vi "2. String retrieve Rulers.vi"() -> ()   [LabVIEW 2017]
uses:
  d59d594f-6358-4fe9-a0ea-ade5f599e91a.vi
  177f037c-d6c1-4684-97ba-f775e359171c.vi
  f8914412-5770-4d7c-8ed9-34d3b6c64140.vi
  83982d16-e29d-493a-892c-93b6b063dd3a.vi
  40fc1cc9-77e3-4a14-9bb9-de70462c7f35.vi
  81b41104-5ca5-45e9-a143-87b761583821.vi
  38ed8c4c-bfe5-4ceb-af5c-8de10cee5e52.vi
  a345cc07-d10f-4275-8a18-17707c3f89e9.vi
  cabc4c38-4671-4b03-9489-31c074b0dc0c.vi
  efc68658-e21b-4998-9bfe-a9de0054dd82.vi
  0842be61-58c2-4c06-9355-20aaf40be817.vi
  a49a9376-e1ff-4fda-bff8-7fdb6b491f6f.vi
  API-String-Arugments-Support/_Support/Convert API String Arguments to Data(variant).vi
panel:
  out "output cluster 11":T1={"Empty API String"="", "2D DBL"=[[3.12, 4.113, 2.3, 5.0, 5.0, 2.3, 4.11, 5.0]], "Retrieved Data"=[[3.12, 4.113, 2.3, 5.0, 5.0, 2.3, 4.11, 5.0]]}
  out "output cluster 10":T2={"Empty API String"="", "Cluster Array"=[{"Name"="", "Child"={"Name"="ddd"}, "Bool"=FALSE}, {"Name"="ddd", "Child"={"Name"=""}, "Bool"=TRUE}], "Retrieved Data"=[{"Name"="", "Child"={"Name"="ddd"}, "Bool"=FALSE}, {"Name"="ddd", "Child"={"Name"=""}, "Bool"=TRUE}]}
  out "output cluster 9":T3={"Empty API String"="", "Cluster"={"Name"="abc", "Child"={"Name"="ddd"}, "Bool"=FALSE}, "Retrieved Data"={"Name"="abc", "Child"={"Name"="ddd"}, "Bool"=FALSE}}
  out "output cluster 8":T4={"Empty API String"="", "1D DBL"=[3.12, 4.11, 5.0], "Retrieved Data"=[3.12, 4.11, 5.0]}
  out "output cluster 7":T5={"Empty API String"="", "Enum"=enum."2 - bbbb", "Retrieved Data"=enum."1 - aaaa"}
  out "output cluster 6":T5
  out "output cluster 5":T6={"Empty API String"="", "Enum"=enum."ccccc", "Retrieved Data"=enum."aaaa"}
  out "output cluster 4":T7={"Empty API String"="", "DBL"=3.1415926, "Retrieved Data"=3.1415926}
  out "output cluster 3":T8={"Empty API String"="", "I32"=66, "Retrieved Data"=66}
  out "output cluster 2":T9={"Empty API String"="", "Boolean"=TRUE, "Retrieved Data"=TRUE}
  out "output cluster":T10={"Empty API String"="", "String"="abcd", "Retrieved Data"=""}
  out "output":T11={"Empty API String"="", "Path"=path "C:/ni-rt/data/a/2023.07.25", "Retrieved Data"=path "C:/ni-rt/data/a/2023.07.25"}
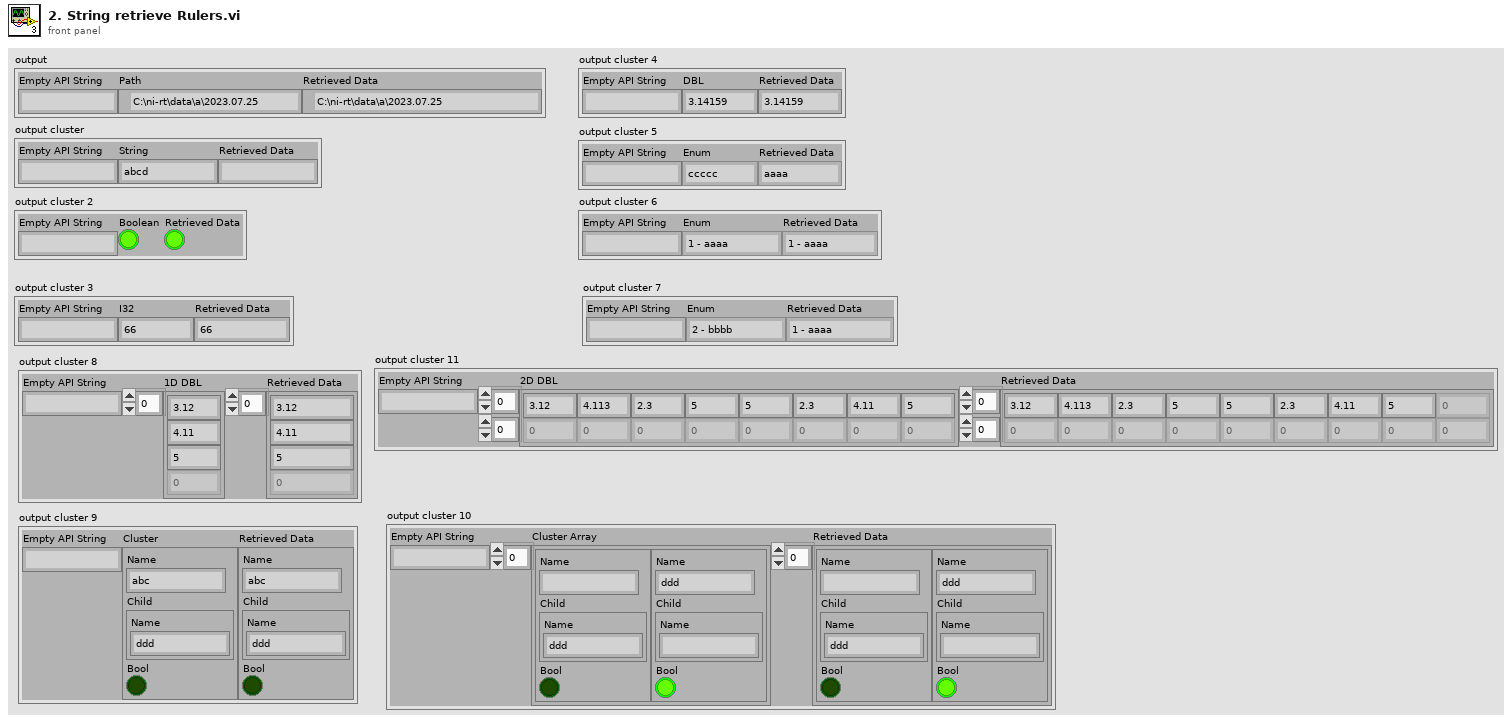
[diagram p1: front panel]
types:
  T1 = cluster{"Empty API String":string, "2D DBL":dbl[][], "Retrieved Data":dbl[][]}
  T2 = cluster{"Empty API String":string, "Cluster Array":cluster{"Name":string, "Child":cluster{"Name":string}, "Bool":bool}[], "Retrieved Data":cluster{"Name":string, "Child":cluster{"Name":string}, "Bool":bool}[]}
  T3 = cluster{"Empty API String":string, "Cluster":cluster{"Name":string, "Child":cluster{"Name":string}, "Bool":bool}, "Retrieved Data":cluster{"Name":string, "Child":cluster{"Name":string}, "Bool":bool}}
  T4 = cluster{"Empty API String":string, "1D DBL":dbl[], "Retrieved Data":dbl[]}
  T5 = cluster{"Empty API String":string, "Enum":enum16{"1 - aaaa", "2 - bbbb", "555 - ccccc"}, "Retrieved Data":enum16{"1 - aaaa", "2 - bbbb", "555 - ccccc"}}
  T6 = cluster{"Empty API String":string, "Enum":enum16{"aaaa", "bbbb", "ccccc"}, "Retrieved Data":enum16{"aaaa", "bbbb", "ccccc"}}
  T7 = cluster{"Empty API String":string, "DBL":dbl, "Retrieved Data":dbl}
  T8 = cluster{"Empty API String":string, "I32":i32, "Retrieved Data":i32}
  T9 = cluster{"Empty API String":string, "Boolean":bool, "Retrieved Data":bool}
  T10 = cluster{"Empty API String":string, "String":string, "Retrieved Data":string}
  T11 = cluster{"Empty API String":string, "Path":path, "Retrieved Data":path}
  T12 = cluster{"Name":string, "Child":cluster{"Name":string}, "Bool":bool}[]
  T13 = cluster{"Name":string, "Child":cluster{"Name":string}, "Bool":bool}
  T14 = cluster{"Empty API String":string, "Data 9":path, "Data":path}
  T15 = cluster{"Empty API String":string, "Data 1":string, "Data":string}
  T16 = cluster{"Empty API String":string, "Data 2":bool, "Data":bool}
  T17 = cluster{"Empty API String":string, "Data 3":i32, "Data":i32}
  T18 = cluster{"Empty API String":string, "Data 4":dbl, "Data":dbl}
  T19 = cluster{"Empty API String":string, "Data 5":enum16{"aaaa", "bbbb", "ccccc"}, "Data":enum16{"aaaa", "bbbb", "ccccc"}}
  T20 = cluster{"Empty API String":string, "Data 6":enum16{"1 - aaaa", "2 - bbbb", "555 - ccccc"}, "Data":enum16{"1 - aaaa", "2 - bbbb", "555 - ccccc"}}
  T21 = cluster{"Empty API String":string, "Data 7":enum16{"1 - aaaa", "2 - bbbb", "555 - ccccc"}, "Data":enum16{"1 - aaaa", "2 - bbbb", "555 - ccccc"}}
  T22 = cluster{"Empty API String":string, "Data 4":dbl[], "Data":dbl[]}
  T23 = cluster{"Empty API String":string, "Data 8":cluster{"Name":string, "Child":cluster{"Name":string}, "Bool":bool}, "Data":cluster{"Name":string, "Child":cluster{"Name":string}, "Bool":bool}}
  T24 = cluster{"Empty API String":string, "Data 10":cluster{"Name":string, "Child":cluster{"Name":string}, "Bool":bool}[], "Data":cluster{"Name":string, "Child":cluster{"Name":string}, "Bool":bool}[]}
  T25 = cluster{"Empty API String":string, "Data 11":dbl[][], "Data":dbl[][]}
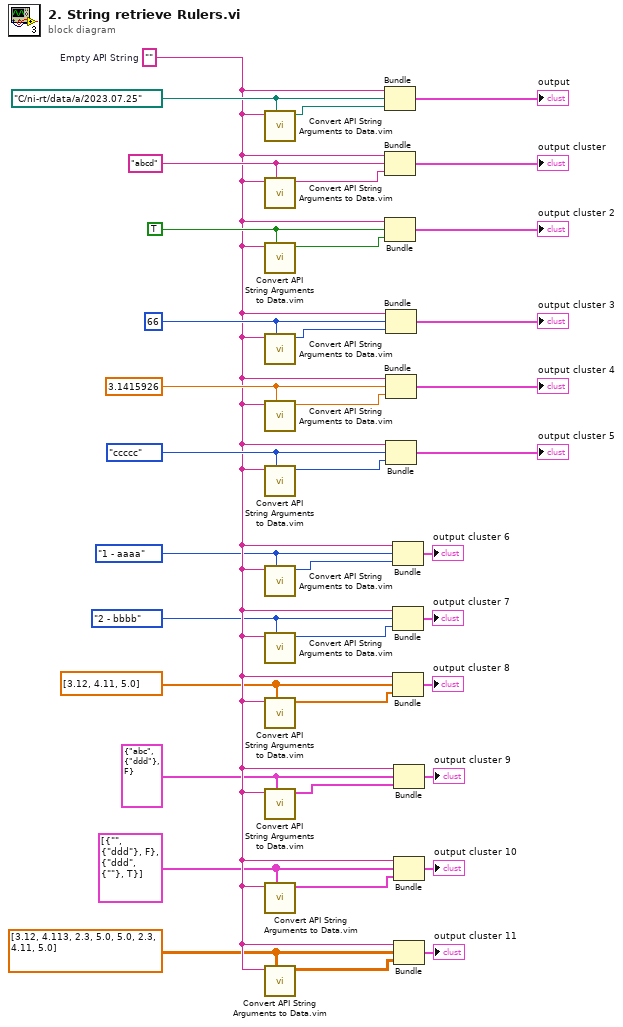
[diagram p0: block diagram]
diagram:
  w7 = dbl[][] [[3.12, 4.113, 2.3, 5.0, 5.0, 2.3, 4.11, 5.0]] ("Data 11")
  w8 = T12 [{"Name"="", "Child"={"Name"="ddd"}, "Bool"=FALSE}, {"Name"="ddd", "Child"={"Name"=""}, "Bool"=TRUE}] ("Data 10")
  w9 = T13 {"Name"="abc", "Child"={"Name"="ddd"}, "Bool"=FALSE} ("Data 8")
  w10 = dbl[] [3.12, 4.11, 5.0] ("Data 4")
  w11 = enum16{"1 - aaaa", "2 - bbbb", "555 - ccccc"}."2 - bbbb" ("Data 7")
  w12 = enum16{"1 - aaaa", "2 - bbbb", "555 - ccccc"}."1 - aaaa" ("Data 6")
  w23 = enum16{"aaaa", "bbbb", "ccccc"}."ccccc" ("Data 5")
  w24 = 3.1415926 ("Data 4")
  w25 = 66 ("Data 3")
  w30 = TRUE ("Data 2")
  w34 = "abcd" ("Data 1")
  w37 = path "C:/ni-rt/data/a/2023.07.25" ("Data 9")
  w13 = ""  # Empty API String
  n1 = call "Convert API String Arguments to Data.vim"("Type"=w37, "String"=w13) -> ("Data"=w36:path)  [unwired: 6 in, 1 out]
  n2 = call "Convert API String Arguments to Data.vim"("Type"=w34, "String"=w13) -> ("Data"=w33:string)  [unwired: 6 in, 1 out]
  n3 = call "Convert API String Arguments to Data.vim"("Type"=w30, "String"=w13) -> ("Data"=w31:bool)  [unwired: 6 in, 1 out]
  n4 = call "Convert API String Arguments to Data.vim"("Type"=w25, "String"=w13) -> ("Data"=w26:i32)  [unwired: 6 in, 1 out]
  n5 = call "Convert API String Arguments to Data.vim"("Type"=w24, "String"=w13) -> ("Data"=w27:dbl)  [unwired: 6 in, 1 out]
  n6 = call "Convert API String Arguments to Data.vim"("Type"=w23, "String"=w13) -> ("Data"=w28:enum16{"aaaa", "bbbb", "ccccc"})  [unwired: 6 in, 1 out]
  n7 = call "Convert API String Arguments to Data.vim"("Type"=w12, "String"=w13) -> ("Data"=w14:enum16{"1 - aaaa", "2 - bbbb", "555 - ccccc"})  [unwired: 6 in, 1 out]
  n8 = call "Convert API String Arguments to Data.vim"("Type"=w11, "String"=w13) -> ("Data"=w15:enum16{"1 - aaaa", "2 - bbbb", "555 - ccccc"})  [unwired: 6 in, 1 out]
  n9 = call "Convert API String Arguments to Data.vim"("Type"=w10, "String"=w13) -> ("Data"=w16:dbl[])  [unwired: 6 in, 1 out]
  n10 = call "Convert API String Arguments to Data.vim"("Type"=w9, "String"=w13) -> ("Data"=w19:T13)  [unwired: 6 in, 1 out]
  n11 = call "Convert API String Arguments to Data.vim"("Type"=w8, "String"=w13) -> ("Data"=w18:T12)  [unwired: 6 in, 1 out]
  n12 = call "Convert API String Arguments to Data.vim"("Type"=w7, "String"=w13) -> ("Data"=w17:dbl[][])  [unwired: 6 in, 1 out]
  n13 = Bundle("Empty API String"=w13, "Data 9"=w37, "Data"=w36) -> (→"output":T14)  [unwired: 1 in]
  n14 = Bundle("Empty API String"=w13, "Data 1"=w34, "Data"=w33) -> (→"output cluster":T15)  [unwired: 1 in]
  n15 = Bundle("Empty API String"=w13, "Data 2"=w30, "Data"=w31) -> (→"output cluster 2":T16)  [unwired: 1 in]
  n16 = Bundle("Empty API String"=w13, "Data 3"=w25, "Data"=w26) -> (→"output cluster 3":T17)  [unwired: 1 in]
  n17 = Bundle("Empty API String"=w13, "Data 4"=w24, "Data"=w27) -> (→"output cluster 4":T18)  [unwired: 1 in]
  n18 = Bundle("Empty API String"=w13, "Data 5"=w23, "Data"=w28) -> (→"output cluster 5":T19)  [unwired: 1 in]
  n19 = Bundle("Empty API String"=w13, "Data 6"=w12, "Data"=w14) -> (→"output cluster 6":T20)  [unwired: 1 in]
  n20 = Bundle("Empty API String"=w13, "Data 7"=w11, "Data"=w15) -> (→"output cluster 7":T21)  [unwired: 1 in]
  n21 = Bundle("Empty API String"=w13, "Data 4"=w10, "Data"=w16) -> (→"output cluster 8":T22)  [unwired: 1 in]
  n22 = Bundle("Empty API String"=w13, "Data 8"=w9, "Data"=w19) -> (→"output cluster 9":T23)  [unwired: 1 in]
  n23 = Bundle("Empty API String"=w13, "Data 10"=w8, "Data"=w18) -> (→"output cluster 10":T24)  [unwired: 1 in]
  n24 = Bundle("Empty API String"=w13, "Data 11"=w7, "Data"=w17) -> (→"output cluster 11":T25)  [unwired: 1 in]
